vi "Key to Reference.vi"(8 "error in (no error)":errorcluster, 10 "Key":string, 11 "Subpanel in":refnum<class "Subpanel.lvclass">) -> (0 "error out":errorcluster, 2 "Reference":refnum<vi>, 3 "Subpanel out":refnum<class "Subpanel.lvclass">)   [LabVIEW 2019, in "Subpanel.lvclass"]
uses:
  Subpanel.lvclass
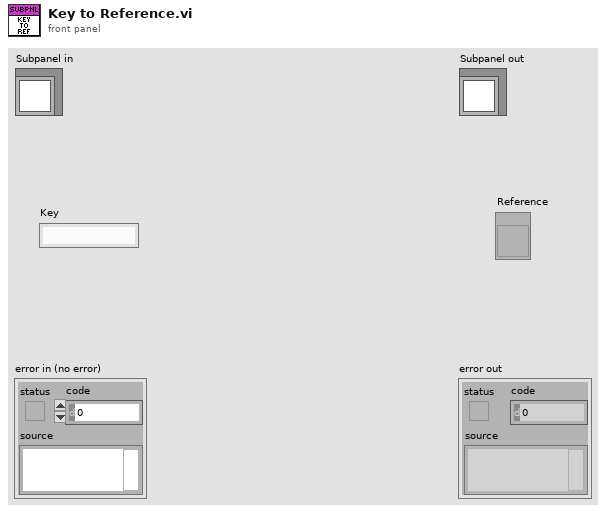
[diagram p1: front panel]
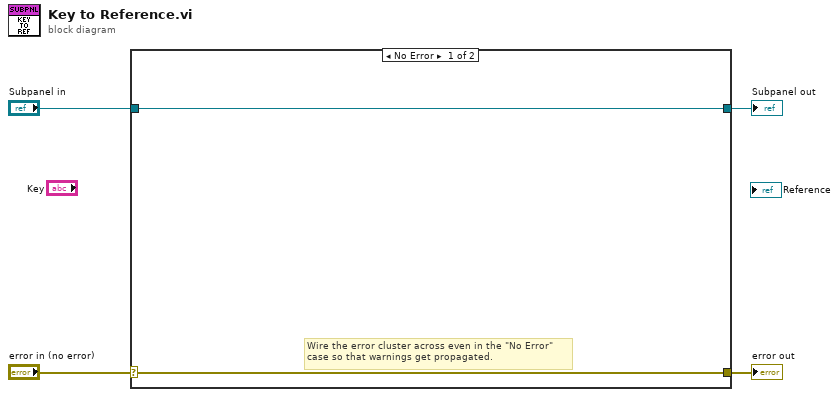
[diagram p0: block diagram]
diagram:
  n1 = case shown="No Error" "error in (no error)" {
    selector: "error in (no error)" -> [w5 w8]
    tunnel: [w5 w8] -> w3
    tunnel: [w6 w7] -> w1
    tunnel: "Subpanel in" -> [w6 w7]
    frame No Error {
      # "Wire the error cluster across even in the \"No Error\"\ncase so that warnings get propagated."
    }
    frame Error {
    }
  }
  "error out" <- w3
  "Subpanel out" <- w1
